vi "Read_Index_File.vi"(0 "Index Filename":path, 1 "Incremental Update?":bool) -> (2 "Filenames":path[](array[path]), 3 "No of Sub vis":string[](array[string]), 4 "Modification times":string[](array[string]))   [LabVIEW 2010]
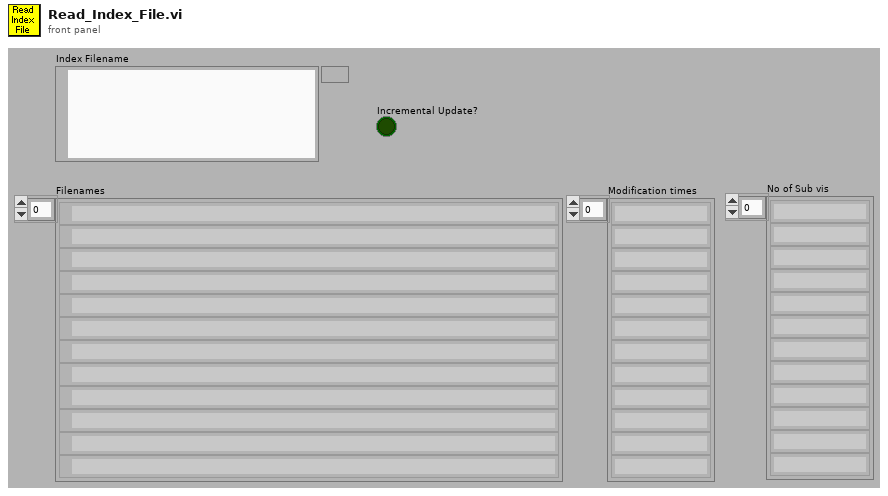
[diagram p1: front panel]
types:
  T1 = enum16{"read/write", "read-only", "write-only", "write-only (truncate)"}
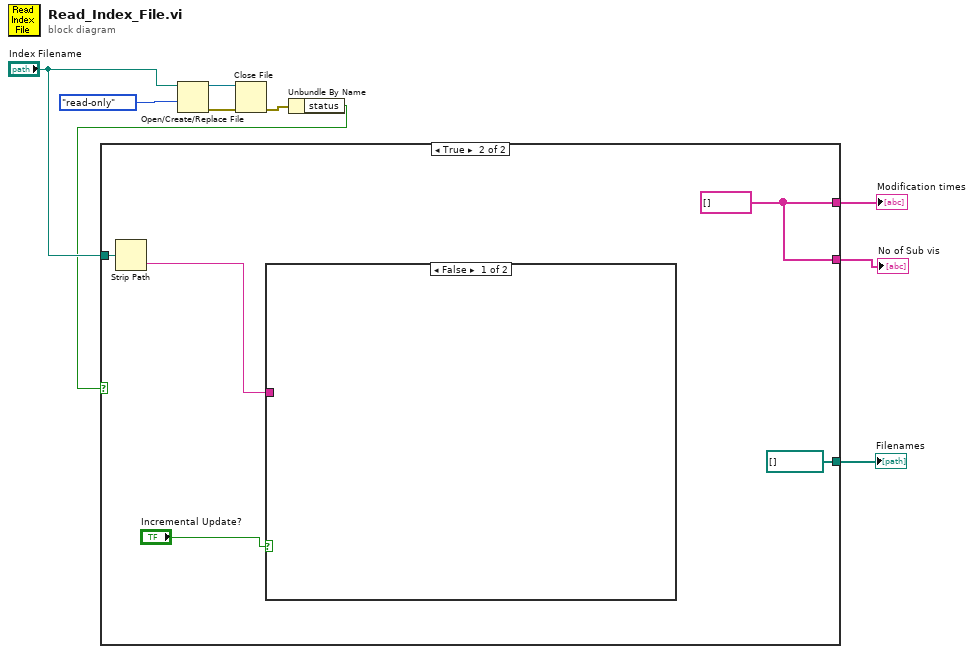
[diagram p0: block diagram]
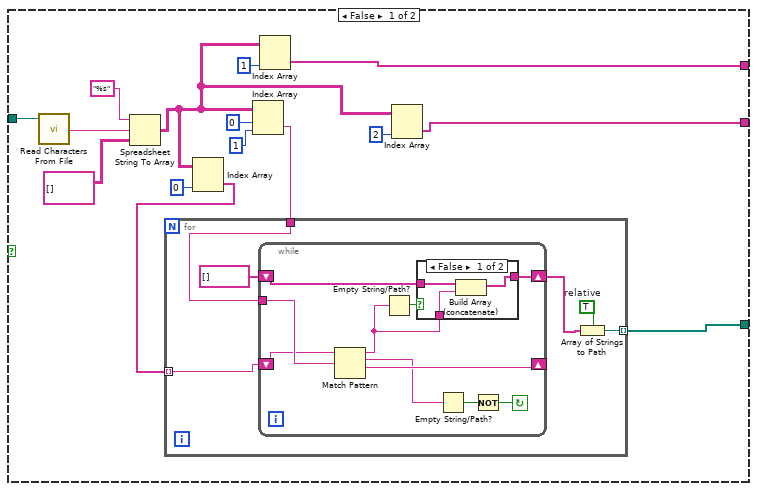
[diagram p2: hidden frame]
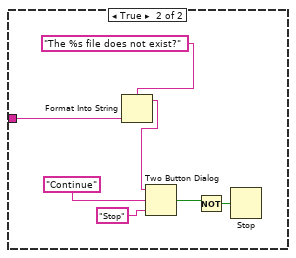
[diagram p4: hidden frame]
diagram:
  n1 = Open/Create/Replace File(file path (use dialog)="Index Filename", access (0:read/write)=T1."read-only" ("open mode (0)")) -> (refnum out=w7:refnum<file>, error out=w4:errorcluster)  [unwired: 1 in, 4 out]
  n2 = Close File(refnum=w7, error in=w4) -> (error out=w5:errorcluster)  [unwired: 1 out]
  n3 = Unbundle By Name(w5) -> ("status"=w1:bool)
  n4 = case shown="True" w1 {
    tunnel: [w10 path[] []] -> w9
    tunnel: [w12 w48] -> w8
    tunnel: "Index Filename" -> [w15 w47]
    tunnel: [w11 w48] -> w2
    frame False {
      n5 = call <vilib>:"Read Characters From File.vi"("file path (dialog if empty)"=w15) -> ("character string"=w17:string)  [unwired: 1 in, 7 out]
      n6 = Spreadsheet String To Array(format string="%s", spreadsheet string=w17, array type (2D Dbl)=string[][] [] ("directory names")) -> (array=w13:string[][])  [unwired: 1 out]
      n7 = Index Array(array=w13, index (col)=0 ("disabled index (col)")) -> (element=w22:string[])  [unwired: 1 in]
      n8 = Index Array(array=w13, index (row)=0, index (col)=1 ("disabled index (col)")) -> (element=w23:string)
      n9 = for {
        tunnel: w22 -> [w29] mode=indexing
        tunnel: w23 -> [w28]
        tunnel: [w25] -> w10 mode=indexing
        w27 = TRUE  # relative
        n10 = while {
          shift-left: string[] [] -> [w33]
          shift-right: [w32] -> w26
          shift-left: w29 -> [w39]
          shift-right: [w38] -> _
          tunnel: w28 -> [w40]
          stop <- w35 continue-if-true
          n11 = Match Pattern(string=w39, regular expression=w40) -> (before substring=w31:string, match substring=w37:string, after substring=w38:string)  [unwired: 2 out]
          n12 = Empty String/Path?(string/path=w31) -> (empty?=w34:bool)
          n13 = case shown="False" w34 {
            tunnel: w33 -> [w43 w44]
            tunnel: [w42 w44] -> w32
            tunnel: w31 -> [w41 _]
            frame False {
              n14 = Build Array (concatenate)(w43, w41) -> (w42:string[])
            }
            frame True {
            }
          }
          n15 = Empty String/Path?(string/path=w37) -> (empty?=w36:bool)
          n16 = Not(x=w36) -> (.not. x?=w35:bool)
        }
        n17 = Array of Strings to Path(0:w26, 1:w27) -> (2:w25:path)
      }
      n18 = Index Array(array=w13, index (col)=1 ("disabled index (col)")) -> (element=w12:string[])  [unwired: 1 in]
      n19 = Index Array(array=w13, index (col)=2 ("disabled index (col)")) -> (element=w11:string[])  [unwired: 1 in]
    }
    frame True {
      w48 = string[] []
      n20 = Strip Path(path=w47) -> (name=w46:string)  [unwired: 1 out]
      n21 = case shown="False" "Incremental Update?" {
        tunnel: w46 -> [_ w52]
        frame False {
        }
        frame True {
          n22 = Format Into String(format string="The %s file does not exist?" ("message"), w52) -> (resulting string=w50:string)  [unwired: 2 in, 1 out]
          n23 = Two Button Dialog(message=w50, 1:"Stop" ("button name (\"OK\")"), 2:"Continue" ("T button name (\"OK\")")) -> (T button?=w54:bool)
          n24 = Not(x=w54) -> (.not. x?=w53:bool)
          n25 = Stop(stop? (T)=w53) -> ()
        }
      }
    }
  }
  "Modification times" <- w8
  "Filenames" <- w9
  "No of Sub vis" <- w2
